vi "Parks-McClellan.vi"(3 "filter type":enum32{"Multiband", "Differentiator", "Hilbert"}(ring), 4 "Band Parameters":T1(array[cluster])=[{"Amplitude"=1.0, "Lower Freq"=0.0, "Higher Freq"=0.2, "Weighted\nRipple"=1.0}, {"Amplitude"=0.0, "Lower Freq"=0.25, "Higher Freq"=0.5, "Weighted\nRipple"=1.0}] {"Weighted\nRipple" min=-1e-308 max=1e+308 format="%0.2e"; "Higher Freq" min=-1e-308 max=1e+308 format="%0.2f"; "Lower Freq" min=-1e-308 max=1e+308 format="%0.2f"; "Amplitude" min=-1e-308 max=1e+308 format="%0.2f"}, 5 "sampling freq: fs":dbl=1.0 min=-1e-308 max=1e+308 format="%0.2f", 6 "# of taps":i32=32) -> (0 "error":i32, 1 "ripple":dbl format="%0.2f", 2 "h":dbl[](array[numeric]))   [LabVIEW 2018, in "NI_AALBase.lvlib"]
doc: "Generates a set of linear-phase FIR multiband digital filter coefficients using the <B># of taps</B>, <B>sampling frequency: fs</B>, <B>Band Parameters</B>, and <B>filter type</B>."
uses:
  NI_AALBase.lvlib
  <resource>/lvanlys.dll
panel:
  # "Parks-McClellan"
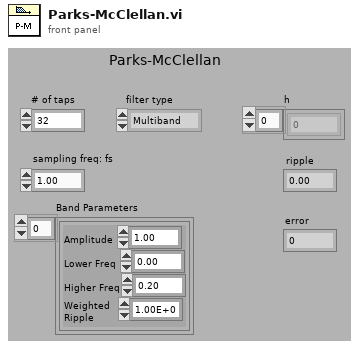
[diagram p1: front panel]
types:
  T1 = cluster{"Amplitude":dbl, "Lower Freq":dbl, "Higher Freq":dbl, "Weighted\nRipple":dbl}[]
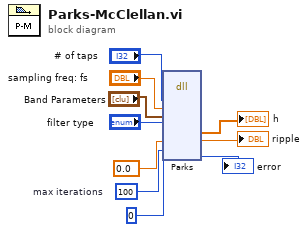
[diagram p0: block diagram]
diagram:
  w8 = 100  # max iterations
  n1 = dll-call lib="C:/Program Files (x86)/National Instruments/LabVIEW 2018/resource/lvanlys.*" fn="Parks"("# of taps"="# of taps", "sampling freq: fs"="sampling freq: fs", "Band Parameters"="Band Parameters", "filter type"="filter type", "output param"=0.0, "max iterations"=w8, "output param"=0) -> ("h"=→"h":dbl[], "output param"=→"ripple":dbl, "output param"=→"error":i32)  [unwired: 10 in, 2 out]
